vi "Get Oil Pump RPM.vi"(0 "Session Handle in":T1, 11 "error in (no error)":errorcluster) -> (4 "Session Handle out":T1, 8 "Success?":bool, 10 "RPM":dbl, 15 "error out":errorcluster)   [LabVIEW 2015, in "Oil.lvclass"]
uses:
  Oil.lvclass
  Typedefs/Session Handle.ctl
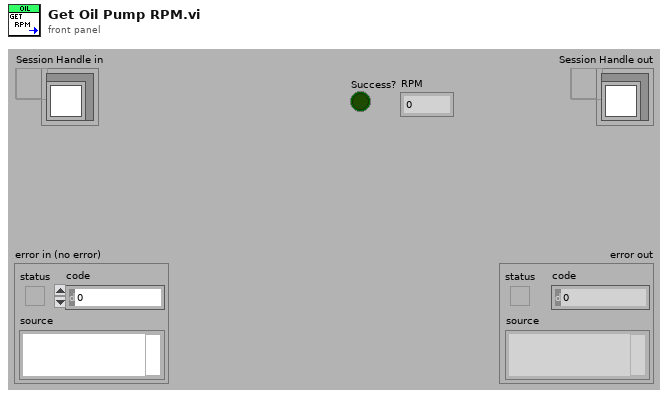
[diagram p1: front panel]
types:
  T1 = typedef "Oil.lvclass/Session Handle.ctl" = refnum<data-value>
  T2 = typedef "XNET Frame CAN.ctl" = cluster{"timestamp":timestamp, "payload":u8[], "identifier":u32, "type":T3, "extended?":bool, "echo?":bool}
  T3 = typedef "XNET Frame Type CAN.ctl" = u8
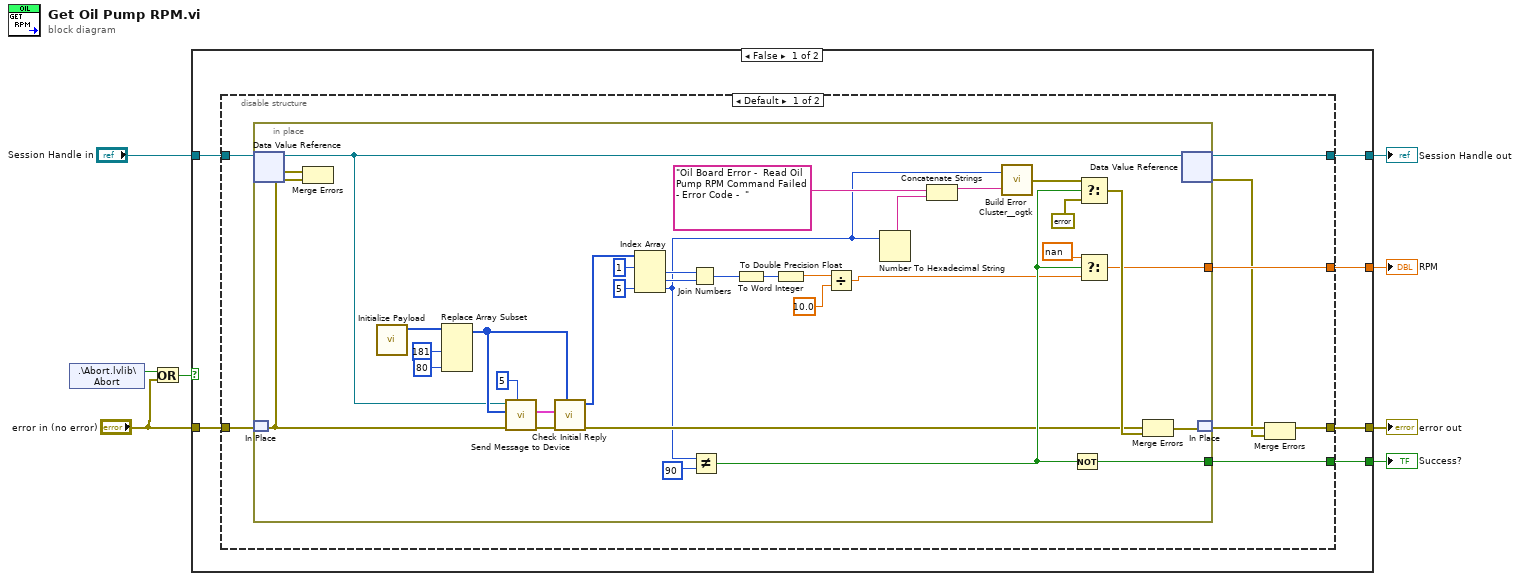
[diagram p0: block diagram]
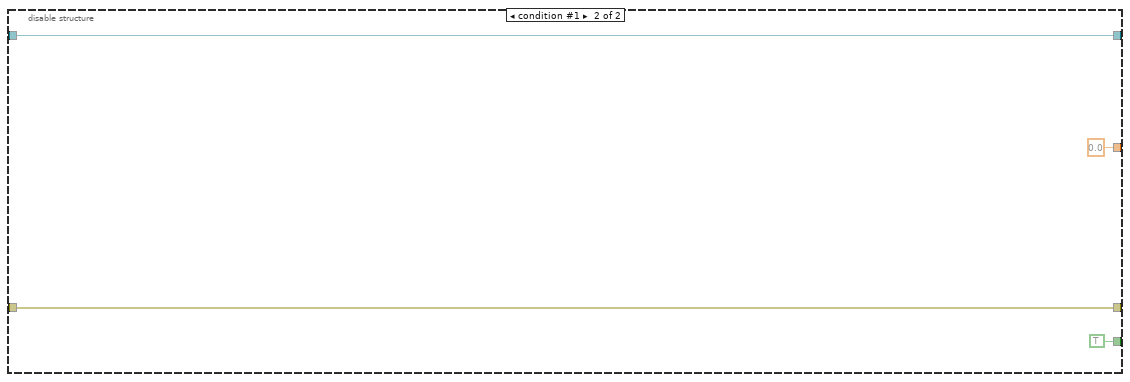
[diagram p2: hidden frame]
diagram:
  n1 = shared-variable ".\\Abort.lvlib\\Abort"() -> (w3:bool)  [unwired: 1 in, 1 out]
  n2 = Or(x=w3, y="error in (no error)") -> (x .or. y?=w2:bool)
  n3 = case shown="False" w2 {
    tunnel: "Session Handle in" -> [w14 w62]
    tunnel: [w13 w62] -> w7
    tunnel: [w12 w61] -> w6
    tunnel: [w11 _] -> w5
    tunnel: [w10 _] -> w4
    tunnel: "error in (no error)" -> [w9 w61]
    frame False {
      n4 = disable-structure shown="Default" {
        disable-tunnel: w14 -> [w22 w60]
        disable-tunnel: [w21 w60] -> w13
        disable-tunnel: [w20 w59] -> w12
        disable-tunnel: [w19 0.0 ("t")] -> w11
        disable-tunnel: [w16 TRUE] -> w10
        disable-tunnel: w9 -> [w15 w59]
        frame condition #0 (active) {
          n5 = in-place {
            in-place-border: [w26] -> w19
            in-place-border: [w31] -> w16
            n6 = in-place-dvr #1(w22) -> (w49:refnum<class "Oil.lvclass">, w56:errorcluster)
            n7 = in-place-match #2(w15) -> (w50:errorcluster)
            n8 = Merge Errors(w50, w56) -> ()  [unwired: 1 out]
            n9 = call "Initialize Payload.vi"() -> ("Initial Payload"=w55:u8[])  [unwired: 11 in]
            n10 = Replace Array Subset(array=w55, new element #1=u8 181 ("new element/subarray"), new element #2=u8 80 ("new element/subarray")) -> (w51:u8[])  [unwired: 2 in]
            n11 = call "Send Message to Device.vi"("Number of Retries"=5, "error in (no error)"=w50, "payload"=w51, "CAN Comm In"=w49) -> ("error out"=w29:errorcluster, "Reply"=w52:T2[])  [unwired: 5 in, 1 out]
            n12 = call "Check Initial Reply.vi"("Write Message"=w51, "error in (no error)"=w29, "Reply"=w52) -> ("error out"=w28:errorcluster, "Data Packet 2"=w48:u8[])  [unwired: 5 in, 2 out]
            n13 = Index Array(array=w48, index #1=1 ("index"), index #3=5 ("index")) -> (element #1=w41:u8, element #2=w40:u8, element #3=w27:u8)  [unwired: 1 in]
            n14 = Join Numbers(hi=w41, lo=w40) -> ((hi.lo)=w43:u16)
            n15 = Not Equal?(x=w27, y=u8 90 ("new element/subarray")) -> (x != y?=w32:bool)
            n16 = To Word Integer(number=w43) -> (16bit integer=w42:i16)
            n17 = To Double Precision Float(number=w42) -> (double precision float=w25:dbl)
            n18 = Divide(x=w25, y=10.0) -> (x/y=w23:dbl)
            n19 = Number To Hexadecimal String(2:w27) -> (0:w36:string)  [unwired: 1 in]
            n20 = Concatenate Strings("Oil Board Error -  Read Oil Pump RPM Command Failed - Error Code -  " ("string"), w36) -> (w39:string)
            n21 = call <userlib>:"Build Error Cluster__ogtk.vi"("String to Prepend to source (\"\")"=w39, "code"=w27) -> ("error out"=w38:errorcluster)
            n22 = Not(x=w32) -> (.not. x?=w31:bool)
            n23 = Select(t=w38, s=w32, f=errorcluster {"status"=FALSE, "code"=0, "source"=""}) -> (s? t:f=w30:errorcluster)
            n24 = Select(t=nan, s=w32, f=w23) -> (s? t:f=w26:dbl)
            n25 = Merge Errors(w28, w30) -> (w34:errorcluster)
            n26 = in-place-dvr #1(w49) -> (w21:T1, w17:errorcluster)
            n27 = in-place-match #2(w34) -> (w18:errorcluster)
          }
          n28 = Merge Errors(w18, w17) -> (w20:errorcluster)
        }
        frame condition #1 {
        }
      }
    }
    frame True {
    }
  }
  "Session Handle out" <- w7
  "error out" <- w6
  "Success?" <- w4
  "RPM" <- w5
